vi "WriteReport.vi"(7 "Diag_Ver":string, 8 "error in (no error)":errorcluster, 9 "StepName":string, 10 "Pass/Fail":bool, 11 "GuiRef":T2={"StringOut"=refnum, "AbortOnFail"=refnum, "SN"=refnum, "SN_Length"=refnum, "TestResult"=refnum, "CycleTime"=refnum, "ErrorCode"=refnum, "UUTStatus"=refnum, "DataBaseEnable?"=refnum, "DUTModel"=refnum, "FixtureID"=refnum, "OperatorID"=refnum, "SNReady"=refnum, "StopSlot"=refnum, "NextStep"=refnum, "PassYeild"=refnum, "Failed"=refnum, "Passed"=refnum, "Tested"=refnum, "TestItemsCtl"={"StepName"="", "TestEnable"=FALSE, "LoopCount"=0, "StopOnFail"=FALSE, "Index"=0, "TestName"="", "通道"="", "参数"="", "TimeStart"=0}, "ProcessBar"=refnum, "Slot"=enum."Slot1", "Row"=3, "States"=refnum, "TestMode"=refnum, "循环次数-DUT"=refnum, "波形图"=refnum, "产品型号"=refnum, "子面板"=refnum, "测试失败项目"=refnum, "测试结果"=refnum, "DUT"=refnum, "Starttime"=refnum, "SlotReady"=refnum, "版本信息"=refnum}) -> (0 "error out":errorcluster caption="error out (no error)", 1 "DBresult":bool, 3 "TestData-NHLD":string[](array[string]))   [LabVIEW 2013]
uses:
  SysControl/Reference.ctl
  SysControl/TestItemsCTL.ctl
  SysControl/Slot.ctl
  SourceCode/CCID info.ctl
  SourceCode/GlobalValue.vi
  <vilib>/Utility/file.llb/Write To Spreadsheet File (string).vi
panel:
  out "Slot":T1
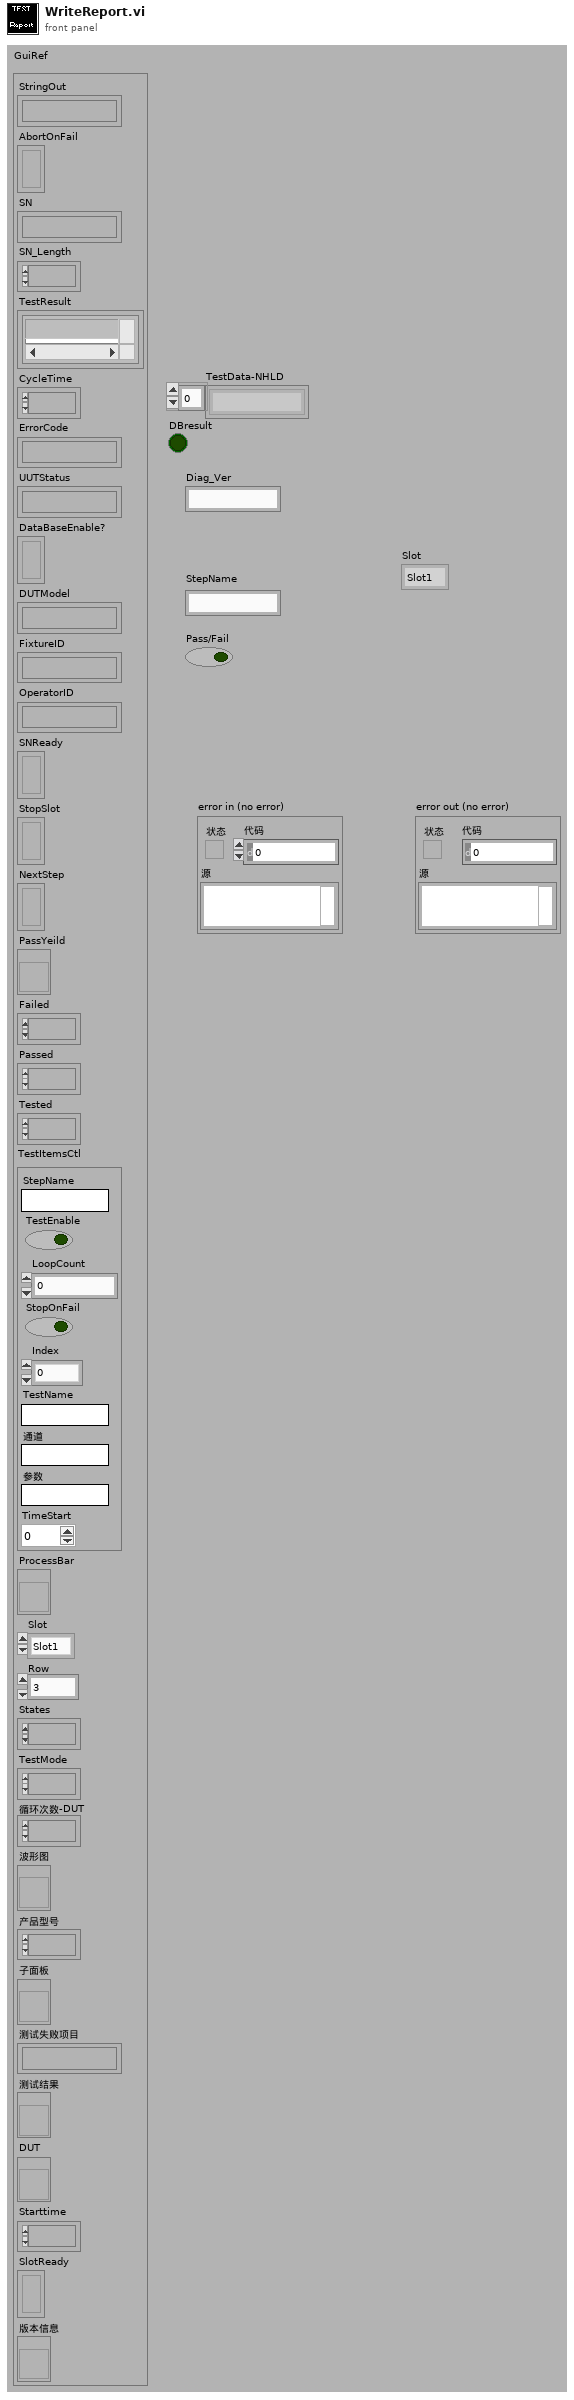
[diagram p1: front panel]
types:
  T1 = typedef "Slot.ctl" = enum16{"Slot1", "Slot2", "Slot3", "Slot4"}
  T2 = typedef "Reference.ctl" = cluster{"StringOut":refnum<vi>, "AbortOnFail":refnum<vi>, "SN":refnum<vi>, "SN_Length":refnum<vi>, "TestResult":refnum<vi>, "CycleTime":refnum<vi>, "ErrorCode":refnum<vi>, "UUTStatus":refnum<vi>, "DataBaseEnable?":refnum<vi>, "DUTModel":refnum<vi>, "FixtureID":refnum<vi>, "OperatorID":refnum<vi>, "SNReady":refnum<vi>, "StopSlot":refnum<vi>, "NextStep":refnum<vi>, "PassYeild":refnum<vi>, "Failed":refnum<vi>, "Passed":refnum<vi>, "Tested":refnum<vi>, "TestItemsCtl":T3, "ProcessBar":refnum<vi>, "Slot":T1, "Row":u32, "States":refnum<vi>, "TestMode":refnum<vi>, "循环次数-DUT":refnum<vi>, "波形图":refnum<vi>, "产品型号":refnum<vi>, "子面板":refnum<vi>, "测试失败项目":refnum<vi>, "测试结果":refnum<vi>, "DUT":refnum<vi>, "Starttime":refnum<vi>, "SlotReady":refnum<vi>, "版本信息":refnum<vi>}
  T3 = typedef "TestItemsCTL.ctl" = cluster{"StepName":string, "TestEnable":bool, "LoopCount":i32, "StopOnFail":bool, "Index":u32, "TestName":string, "通道":string, "参数":string, "TimeStart":u32}
  T4 = typedef "CCID info.ctl" = enum16{"Fw Ver", "HW Ver", "CCID", "WiFiName", "DevID"}
  T5 = enum16{"open", "replace", "create", "open or create", "replace or create", "replace or create with confirmation"}
  T6 = enum16{"Production Mode", "Selection Mode", "Debug Mode", "Loop Mode", "Stop Test"}
  T7 = cluster{"Serial#":string, "TestDate_Time":string, "Operator":string, "TestStation":string, "Fixture#":string, "TestTime":string, "Diag_Ver":string, "Pass_Fail":string}
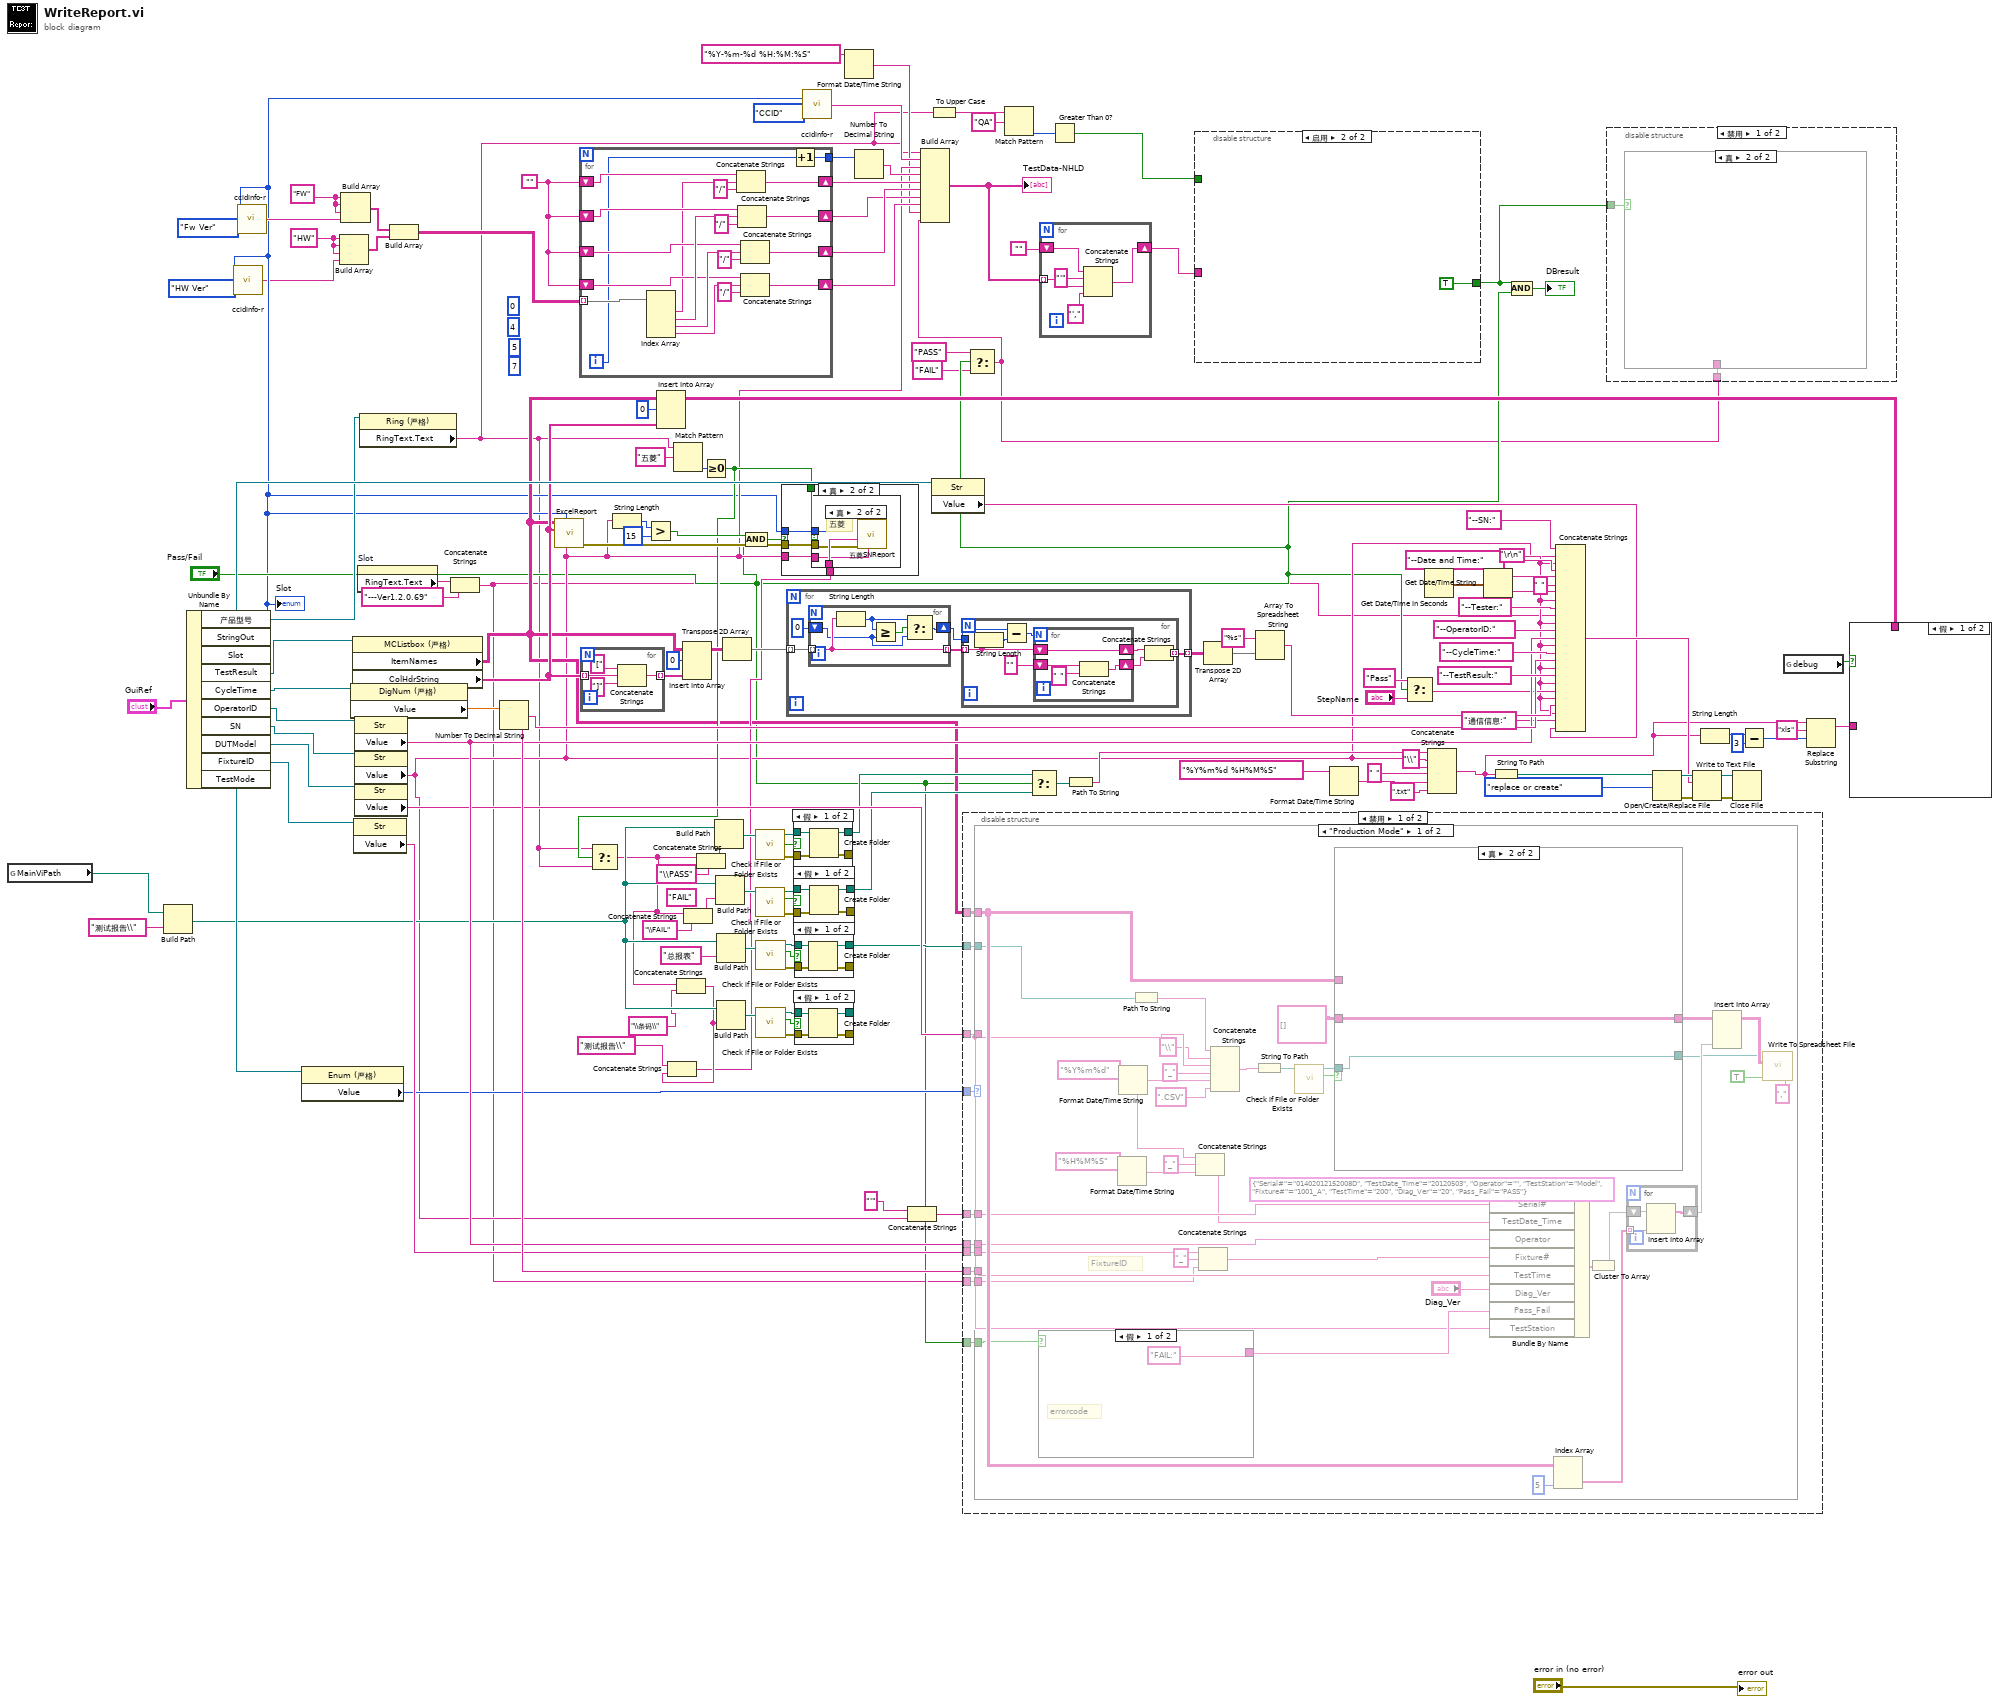
[diagram p0: block diagram]
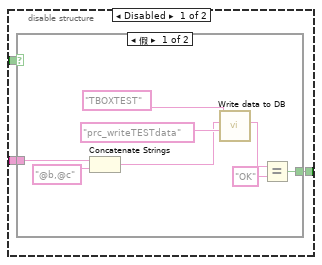
[diagram p2: hidden frame]
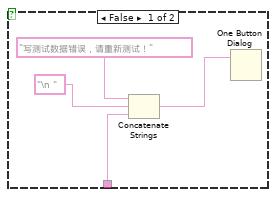
[diagram p4: hidden frame]
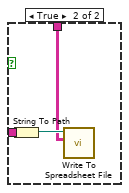
[diagram p6: hidden frame]
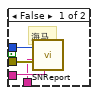
[diagram p8: hidden frame]
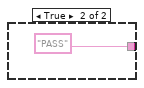
[diagram p10: hidden frame]
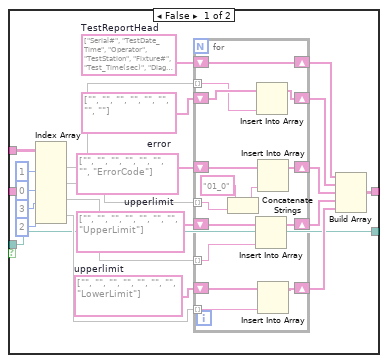
[diagram p11: hidden frame]
diagram:
  (unwired) 7 ("索引")
  (unwired) 5 ("索引")
  (unwired) 4 ("索引")
  (unwired) 0 ("索引")
  w12 = "HW"
  w13 = "FW"
  w39 = ""
  (unwired) "FAIL" ("name or relative path")
  w80 = "\r\n"
  n1 = global read "GlobalValue.vi" "MainViPath"() -> (w74:path)
  n2 = Build Path(base path=w74, name or relative path="测试报告\\" ("名称或相对路径")) -> (appended path=w69:path)
  n3 = Unbundle By Name("GuiRef") -> ("产品型号"=w63:refnum<vi>, "StringOut"=w76:refnum<vi>, "Slot"=w18:T1, "TestResult"=w114:refnum<vi>, "CycleTime"=w113:refnum<vi>, "OperatorID"=w112:refnum<vi>, "SN"=w111:refnum<vi>, "DUTModel"=w110:refnum<vi>, "FixtureID"=w105:refnum<vi>, "TestMode"=w83:refnum<vi>)
  "Slot" <- w18
  n4 = call "ccidinfo-r.vi"("Data Type"=CCID_info."HW Ver", "Slot"=w18) -> ("Data"=w17:string)
  n5 = call "ccidinfo-r.vi"("Data Type"=CCID_info."Fw Ver", "Slot"=w18) -> ("Data"=w19:string)
  n6 = property class="Enum (严格)"(reference=w83) -> ("Value"=w82:T6)  [unwired: 1 in, 2 out]
  n7 = Build Array(w12, w12, w12, w17) -> (w15:string[])
  n8 = Build Array(w13, w13, w13, w19) -> (w16:string[])
  n9 = property class="DigNum (严格)"(reference=w113) -> ("Value"=w109:dbl)  [unwired: 1 in, 2 out]
  n10 = property class="MCListbox (严格)"(reference=w114) -> ("ItemNames"=w40:string[][], "ColHdrString"=w44:string[])  [unwired: 1 in, 2 out]
  n11 = property class="Str"(reference=w105) -> ("Value"=w104:string)  [unwired: 1 in, 2 out]
  n12 = property class="Str"(reference=w112) -> ("Value"=w108:string)  [unwired: 1 in, 2 out]
  n13 = property class="Str"(reference=w111) -> ("Value"=w32:string)  [unwired: 1 in, 2 out]
  n14 = property class="Str"(reference=w110) -> ("Value"=w107:string)  [unwired: 1 in, 2 out]
  n15 = property on="Slot" class="Enum (严格)"() -> ("RingText.Text"=w5:string)  [unwired: 2 in, 2 out]
  n16 = property class="Ring (严格)"(reference=w63) -> ("RingText.Text"=w11:string)  [unwired: 1 in, 2 out]
  n17 = Build Array(w16, w15) -> (w14:string[][])
  n18 = Concatenate Strings(w5, "---Ver1.2.0.69" ("字符串")) -> (w3:string)
  n19 = Number To Decimal String(number=w109) -> (decimal integer string=w118:string)  [unwired: 1 out]
  n20 = call "ExcelReport.vi"("SN"=w32, "Slot"=w18, "列首字符串"=w44, "TestResults"=w40) -> ("error out"=w68:errorcluster)  [unwired: 7 in]
  n21 = for {
    tunnel: w14 -> [w166] mode=indexing
    shift-right: [w165] -> w38
    shift-left: w39 -> [w164]
    shift-right: [w158] -> w35
    shift-left: w39 -> [w161]
    shift-right: [w156] -> w36
    shift-left: w39 -> [w157]
    shift-right: [w151] -> w37
    shift-left: w39 -> [w153]
    tunnel: [w150] -> w34
    i -> [w149]
    n22 = Index Array(array=w166) -> (element #1=w148:string, element #2=w160:string, element #3=w154:string, element #4=w152:string)  [unwired: 4 in]
    n23 = Concatenate Strings(w164, w148, "/" ("字符串")) -> (w165:string)
    n24 = Concatenate Strings(w161, w160, "/" ("字符串")) -> (w158:string)
    n25 = Concatenate Strings(w157, w154, "/" ("字符串")) -> (w156:string)
    n26 = Concatenate Strings(w153, w152, "/" ("字符串")) -> (w151:string)
    n27 = Increment(x=w149) -> (x+1=w150:i32)
  }
  n28 = for "For循环" {
    tunnel: w44 -> [w169] mode=indexing
    tunnel: [w167] -> w135 mode=indexing
    n29 = Concatenate Strings("[" ("字符串"), w169, "]" ("字符串")) -> (w167:string)
  }
  n30 = String Length(string=w32) -> (length=w67:i32)
  n31 = Greater?(x=w67, y=15) -> (0:w65:bool)
  n32 = Insert Into Array(array=w40, index (row)=0 ("索引 (行)"), new element=w44) -> (w42:string[][])  [unwired: 1 in]
  n33 = Match Pattern(string=w11, regular expression="五菱" ("正则表达式")) -> (offset past match=w61:i32)  [unwired: 1 in, 3 out]
  n34 = Insert Into Array(array=w40, index (row)=0 ("索引 (行)"), new element=w135) -> (w138:string[][])  [unwired: 1 in]
  n35 = Greater Or Equal To 0?(x=w61) -> (x >= 0?=w60:bool)
  n36 = Select(t=w11, s=w60, f=w11) -> (s? t:f=w54:string)
  n37 = Concatenate Strings(w54, "\\条码\\" ("name or relative path")) -> (w52:string)
  n38 = Concatenate Strings("测试报告\\" ("字符串"), w52) -> (w51:string)
  n39 = Concatenate Strings(w54, "\\FAIL" ("name or relative path")) -> (w56:string)
  n40 = Concatenate Strings(w54, "\\PASS" ("name or relative path")) -> (w59:string)
  n41 = Build Path(base path=w69, name or relative path=w59) -> (appended path=w95:path)
  n42 = Build Path(base path=w69, name or relative path=w56) -> (appended path=w94:path)
  n43 = Build Path(base path=w69, name or relative path="总报表") -> (appended path=w102:path)
  n44 = Build Path(base path=w69, name or relative path=w52) -> (appended path=w71:path)
  n45 = Transpose 2D Array(2D array=w138) -> (transposed array=w146:string[][])
  n46 = And(x=w65, y="Pass/Fail") -> (x .and. y?=w64:bool)
  n47 = call <vilib>:"Check if File or Folder Exists.vi"("path"=w95) -> ("error out"=w99:errorcluster, "file or folder exists?"=w85:bool, "dup path"=w98:path)  [unwired: 1 in, 7 out]
  n48 = call <vilib>:"Check if File or Folder Exists.vi"("path"=w94) -> ("error out"=w96:errorcluster, "file or folder exists?"=w84:bool, "dup path"=w97:path)  [unwired: 1 in, 7 out]
  n49 = call <vilib>:"Check if File or Folder Exists.vi"("path"=w102) -> ("error out"=w101:errorcluster, "file or folder exists?"=w86:bool, "dup path"=w103:path)  [unwired: 1 in, 7 out]
  n50 = call <vilib>:"Check if File or Folder Exists.vi"("path"=w71) -> ("error out"=w72:errorcluster, "file or folder exists?"=w73:bool, "dup path"=w70:path)  [unwired: 1 in, 7 out]
  n51 = case shown="真" w64 {
    tunnel: w18 -> [_ w175]
    tunnel: w32 -> [_ w174]
    tunnel: w68 -> [_ w173]
    tunnel: w60 -> [_ w172]
    tunnel: w51 -> [_ w171]
    frame False {
    }
    frame True {
      n52 = case shown="真" w172 {
        tunnel: w175 -> [w179 w180]
        tunnel: w174 -> [w178 w182]
        tunnel: w173 -> [w177 w181]
        tunnel: w171 -> [w176 w183]
        frame False {
          # "海马"
          n53 = call "SNReport.vi"("SN"=w178, "Slot"=w179, "error in (no error)"=w177, "字符串"=w176) -> ()  [unwired: 7 in, 1 out]
        }
        frame True {
          # "五菱"
          n54 = call "五菱SNReport.vi"("SN"=w182, "Slot"=w180, "error in (no error)"=w181, "字符串"=w183) -> ()  [unwired: 7 in, 1 out]
        }
      }
    }
  }
  n55 = for "For循环" {
    tunnel: w146 -> [w186] mode=indexing
    tunnel: [w185] -> w145 mode=indexing
    n56 = for "For循环" {
      tunnel: w186 -> [w205] mode=indexing
      shift-right: [w201] -> w184
      shift-left: 0 -> [w203]
      tunnel: [w205] -> w187 mode=indexing
      n57 = String Length(string=w205) -> (length=w204:i32)
      n58 = Greater Or Equal?(x=w204, y=w203) -> (x >= y?=w202:bool)
      n59 = Select(t=w204, s=w202, f=w203) -> (s? t:f=w201:i32)
    }
    n60 = for "For循环" {
      tunnel: w187 -> [w189] mode=indexing
      tunnel: [w194] -> w185 mode=indexing
      tunnel: w184 -> [w192]
      n61 = String Length(string=w189) -> (length=w196:i32)
      n62 = Subtract(x=w192, y=w196) -> (x-y=w195:i32)
      n63 = for "For循环" {
        N: w195 -> [_]
        shift-right: [w198] -> w191
        shift-left: "" -> [w199]
        shift-right: [w197] -> w190
        shift-left: w189 -> [w197]
        n64 = Concatenate Strings(w199, " ") -> (w198:string)
      }
      n65 = Concatenate Strings(w190, w191) -> (w194:string)
    }
  }
  n66 = case shown="假" w85 {
    tunnel: w98 -> [w209 w210]
    tunnel: [w208 _] -> _
    tunnel: w99 -> [w207 _]
    tunnel: [w206 w210] -> w90
    frame False {
      n67 = Create Folder(path (use dialog)=w209, error in=w207) -> (created path=w206:path, error out=w208:errorcluster)  [unwired: 2 out]
    }
    frame True {
    }
  }
  n68 = case shown="假" w84 {
    tunnel: w97 -> [w214 w215]
    tunnel: [w213 _] -> _
    tunnel: w96 -> [w212 _]
    tunnel: [w211 w215] -> w89
    frame False {
      n69 = Create Folder(path (use dialog)=w214, error in=w212) -> (created path=w211:path, error out=w213:errorcluster)  [unwired: 2 out]
    }
    frame True {
    }
  }
  n70 = case shown="假" w86 {
    tunnel: w103 -> [w219 w220]
    tunnel: [w218 _] -> _
    tunnel: w101 -> [w217 _]
    tunnel: [w216 w220] -> w100
    frame False {
      n71 = Create Folder(path (use dialog)=w219, error in=w217) -> (created path=w216:path, error out=w218:errorcluster)  [unwired: 2 out]
    }
    frame True {
    }
  }
  n72 = case shown="假" w73 {
    tunnel: w70 -> [w224 w225]
    tunnel: [w223 _] -> _
    tunnel: w72 -> [w222 _]
    tunnel: [w221 w225] -> _
    frame False {
      n73 = Create Folder(path (use dialog)=w224, error in=w222) -> (created path=w221:path, error out=w223:errorcluster)  [unwired: 2 out]
    }
    frame True {
    }
  }
  n74 = call "ccidinfo-r.vi"("Data Type"=CCID_info."CCID", "Slot"=w18) -> ("Data"=w30:string)
  n75 = Format Date/Time String(time format string (%c)="%Y-%m-%d %H:%M:%S" ("时间格式字符串(%c)")) -> (date/time string=w28:string)  [unwired: 2 in]
  n76 = Number To Decimal String(number=w34) -> (decimal integer string=w33:string)  [unwired: 1 in]
  n77 = Concatenate Strings("'" ("string"), w32) -> (w116:string)
  n78 = To Upper Case(1:w11) -> (0:w10:string)
  n79 = property class="Str"(reference=w76) -> ("Value"=w75:string)  [unwired: 1 in, 2 out]
  n80 = disable-structure shown="禁用" {
    disable-tunnel: w118 -> [w235 _]
    disable-tunnel: w116 -> [w234 _]
    disable-tunnel: w3 -> [w233 _]
    disable-tunnel: w40 -> [w232 _]
    disable-tunnel: w108 -> [w231 _]
    disable-tunnel: w107 -> [w230 _]
    disable-tunnel: w104 -> [w229 _]
    disable-tunnel: w100 -> [w228 _]
    disable-tunnel: w82 -> [w227 _]
    disable-tunnel: "Pass/Fail" -> [w226 _]
    frame Disabled {
      n81 = case shown="\"Production Mode\"" w227 {
        tunnel: w232 -> [w269 _]
        tunnel: w234 -> [w257 _]
        tunnel: w226 -> [w260 _]
        tunnel: w233 -> [w239 _]
        tunnel: w235 -> [w245 _]
        tunnel: w231 -> [w248 _]
        tunnel: w230 -> [w242 _]
        tunnel: w229 -> [w237 _]
        tunnel: w228 -> [w236 _]
        frame "Production Mode" {
          # "FixtureID"
          n82 = case shown="假" w260 {
            tunnel: ["FAIL:" ("TesterID") "PASS" ("TesterID")] -> w243
            frame False {
              # "errorcode"
            }
            frame True {
            }
          }
          n83 = Format Date/Time String(time format string (%c)="%H%M%S") -> (date/time string=w250:string)  [unwired: 2 out]
          n84 = Format Date/Time String(time format string (%c)="%Y%m%d") -> (date/time string=w251:string)  [unwired: 2 out]
          n85 = Path To String(path=w236) -> (string=w240:string)
          n86 = Concatenate Strings(w251, "_" ("string"), w250) -> (w249:string)
          n87 = Concatenate Strings(w237, "_" ("string"), w239) -> (w246:string)
          n88 = Concatenate Strings(w240, "\\" ("字符串"), w242, "_", w251, ".CSV" ("字符串")) -> (w262:string)
          n89 = String To Path(string=w262) -> (path=w255:path)
          n90 = call <vilib>:"Check if File or Folder Exists.vi"("path"=w255) -> ("file or folder exists?"=w266:bool, "dup path"=w254:path)  [unwired: 1 in, 8 out]
          n91 = case shown="真" w266 {
            tunnel: [w295 w314] -> w272
            tunnel: w269 -> [w280 _]
            tunnel: string[][] [] ("数组 2") -> [_ w314]
            tunnel: w254 -> [w277 w313]
            tunnel: [w277 w313] -> w238
            frame False {
              w290 = string[] ["", "", "", "", "", "", "", "LowerLimit"]  # upperlimit
              w292 = string[] ["", "", "", "", "", "", "", "UpperLimit"]  # upperlimit
              w293 = string[] ["", "", "", "", "", "", "", "ErrorCode"]  # error
              w297 = string[] ["Serial#", "TestDate_Time", "Operator", "TestStation", "Fixture#", "Test_Time(sec)", "Diag_Ver", "Pass_Fail", "NAME", ""]  # TestReportHead
              n92 = Index Array(array=w280, index (col) #1=1 ("禁用的索引 (列)"), index (col) #2=0 ("索引 (列)"), index (col) #3=3 ("索引 (列)"), index (col) #4=2 ("索引 (列)")) -> (element #1=w283:string[], element #2=w284:string[], element #3=w279:string[], element #4=w278:string[])  [unwired: 4 in]
              n93 = for {
                shift-right: [w301] -> w296
                shift-left: w297 -> [w301]
                tunnel: w283 -> [w302] mode=indexing
                shift-right: [w311] -> w294
                shift-left: w293 -> [w312]
                tunnel: w284 -> [w299] mode=indexing
                tunnel: w279 -> [w310] mode=indexing
                shift-right: [w308] -> w291
                shift-left: w292 -> [w309]
                shift-right: [w307] -> w289
                shift-left: w290 -> [w306]
                tunnel: w278 -> [w305] mode=indexing
                shift-right: [w303] -> w287
                shift-left: string[] ["", "", "", "", "", "", "", ""] -> [w304]
                n94 = Concatenate Strings("01_0" ("string"), w299) -> (w298:string)
                n95 = Insert Into Array(array=w309, new element=w310) -> (w308:string[])  [unwired: 1 in]
                n96 = Insert Into Array(array=w304, new element=w302) -> (w303:string[])  [unwired: 1 in]
                n97 = Insert Into Array(array=w312, new element=w298) -> (w311:string[])  [unwired: 1 in]
                n98 = Insert Into Array(array=w306, new element=w305) -> (w307:string[])  [unwired: 1 in]
              }
              n99 = Build Array(w296, w287, w294, w291, w289) -> (w295:string[][])
            }
            frame True {
            }
          }
          n100 = Bundle By Name(cluster=T7 {"Serial#"="01402012152008D", "TestDate_Time"="20120503", "Operator"="", "TestStation"="Model", "Fixture#"="1001_A", "TestTime"="200", "Diag_Ver"="20", "Pass_Fail"="PASS"} ("output cluster"), "Serial#"=w257, "TestDate_Time"=w249, "Operator"=w248, "Fixture#"=w246, "TestTime"=w245, "Diag_Ver"="Diag_Ver", "Pass_Fail"=w243, "TestStation"=w242) -> (w259:T7)
          n101 = Index Array(array=w269, index (col)=5 ("索引 (列)")) -> (element=w270:string[])  [unwired: 1 in]
          n102 = Cluster To Array(cluster=w259) -> (array=w274:string[])
          n103 = for {
            tunnel: w270 -> [w316] mode=indexing
            shift-right: [w315] -> w273
            shift-left: w274 -> [w317]
            n104 = Insert Into Array(array=w317, new element=w316) -> (w315:string[])  [unwired: 1 in]
          }
          n105 = Insert Into Array(array=w272, new element=w273) -> (w265:string[][])  [unwired: 2 in]
          n106 = call-poly <vilib>:"Write To Spreadsheet File.vi"("delimiter (\\t)"="," ("delimiter (\\t)"), "append to file? (new file:F)"=TRUE, "2D data"=w265, "file path (dialog if empty)"=w238) -> ()  [unwired: 3 in, 2 out]
        }
        frame "Debug Mode", Default {
        }
      }
    }
    frame Enabled {
    }
  }
  n107 = Select(t="PASS" ("元素"), s="Pass/Fail", f="FAIL" ("元素")) -> (s? t:f=w8:string)
  n108 = Build Array(w11, w30, w32, w33, w38, w36, w35, w37, w28, w8) -> (w27:string[])
  "TestData-NHLD" <- w27
  n109 = Match Pattern(string=w10, regular expression="QA" ("正则表达式")) -> (offset past match=w7:i32)  [unwired: 1 in, 3 out]
  n110 = Select(t=w90, s="Pass/Fail", f=w89) -> (s? t:f=w88:path)
  n111 = for {
    tunnel: w27 -> [w320] mode=indexing
    shift-right: [w318] -> w26
    shift-left: "" -> [w322]
    n112 = Concatenate Strings(w322, "'" ("字符串"), w320, "'," ("字符串")) -> (w318:string)
  }
  n113 = Greater Than 0?(x=w7) -> (x > 0?=w6:bool)
  n114 = Path To String(path=w88) -> (string=w87:string)
  n115 = disable-structure shown="启用" {
    disable-tunnel: w26 -> [w325 _]
    disable-tunnel: w6 -> [w324 _]
    disable-tunnel: [w323 TRUE] -> w1
    frame Disabled {
      n116 = case shown="假" w324 {
        selector: w324 -> [_ w334]
        tunnel: w325 -> [w333 _]
        tunnel: [w332 w334] -> w323
        frame False {
          n117 = Concatenate Strings(w333, "@b,@c" ("元素")) -> (w327:string)
          n118 = call "Write data to DB.vi"("Procedure name"="prc_writeTESTdata", "all string"=w327, "DSN name"="TBOXTEST") -> ("ResultA"=w329:string)  [unwired: 6 in, 2 out]
          n119 = Equal?(x=w329, y="OK") -> (x = y?=w332:bool)
        }
        frame True {
        }
      }
    }
    frame Enabled {
    }
  }
  n120 = Transpose 2D Array(2D array=w145) -> (transposed array=w139:string[][])
  n121 = Array To Spreadsheet String(array=w139, 3:"%s" ("format string")) -> (spreadsheet string=w142:string)  [unwired: 1 out]
  n122 = Format Date/Time String(time format string (%c)="%Y%m%d %H%M%S") -> (date/time string=w128:string)  [unwired: 2 out]
  n123 = Select(t="Pass", s="Pass/Fail", f="StepName") -> (s? t:f=w91:string)
  n124 = Get Date/Time In Seconds() -> (seconds since 1Jan1904=w141:timestamp)
  n125 = Concatenate Strings(w87, "\\" ("string"), w32, " " ("string"), w128, ".txt" ("字符串")) -> (w48:string)
  n126 = Get Date/Time String(seconds (now)=w141) -> (date string=w124:string, time string=w122:string)  [unwired: 2 out]
  n127 = String To Path(string=w48) -> (path=w134:path)
  n128 = And(x=w1, y="Pass/Fail") -> (x .and. y?=→"DBresult":bool)
  n129 = Concatenate Strings("--SN:" ("element"), w32, w80, "--Date and Time:" ("元素"), w124, " " ("字符串"), w122, w80, "--Tester:" ("element"), w3, w80, "--OperatorID:" ("string"), w108, w80, "--CycleTime:" ("字符串"), w118, w80, "--TestResult:" ("元素"), w80, w91, w80, w142, w80, "通信信息:" ("字符串"), w75) -> (w130:string)
  n130 = disable-structure shown="禁用" {
    disable-tunnel: w8 -> [w337 _]
    disable-tunnel: w1 -> [w336 _]
    frame Disabled {
      n131 = case shown="真" w336 {
        tunnel: w337 -> [w339 _]
        frame False {
          n132 = Concatenate Strings("写测试数据错误，请重新测试！" ("消息"), "\n ", w339) -> (w338:string)
          n133 = One Button Dialog(message=w338) -> ()  [unwired: 1 in, 1 out]
        }
        frame True {
        }
      }
    }
    frame Enabled {
    }
  }
  n134 = Open/Create/Replace File(file path (use dialog)=w134, operation (0:open)=T5."replace or create" ("操作(0:open)")) -> (refnum out=w133:refnum<file>, error out=w131:errorcluster)  [unwired: 1 in, 4 out]
  n135 = Write to Text File(file (use dialog)=w133, text=w130, error in=w131) -> (refnum out=w136:refnum<file>, error out=w137:errorcluster)  [unwired: 2 out]
  n136 = String Length(string=w48) -> (length=w50:i32)
  n137 = Close File(refnum=w136, error in=w137) -> ()  [unwired: 2 out]
  n138 = Subtract(x=w50, y=3) -> (x-y=w46:i32)
  n139 = global read "GlobalValue.vi" "debug"() -> (w41:bool)
  n140 = Replace Substring(3:w46, 4:"xls" ("子字符串(\"\")"), 5:w48) -> (1:w45:string)  [unwired: 1 in, 1 out]
  n141 = case shown="假" w41 {
    tunnel: w45 -> [_ w344]
    tunnel: w42 -> [_ w342]
    frame False {
    }
    frame True {
      n142 = String To Path(string=w344) -> (path=w343:path)
      n143 = call-poly <vilib>:"Write To Spreadsheet File.vi"("2D data"=w342, "file path (dialog if empty)"=w343) -> ()  [unwired: 6 in, 1 out]
    }
  }
  "error out" <- "error in (no error)"
